vi "UIEH(ver.StateMachine).vi"() -> ()   [LabVIEW 2023]
panel:
  in  "종료":bool
  in  "저장":bool
  in  "분석":bool
  in  "측정":bool
  out "Count":i32
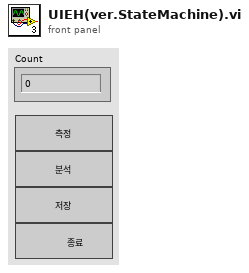
[diagram p1: front panel]
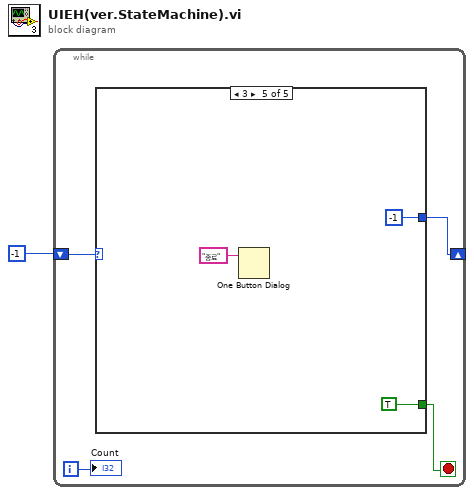
[diagram p0: block diagram]
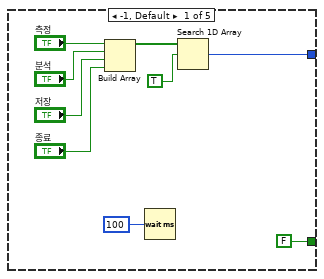
[diagram p2: hidden frame]
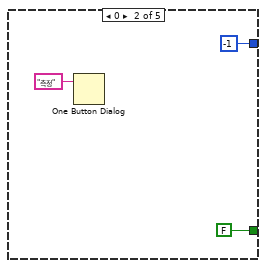
[diagram p3: hidden frame]
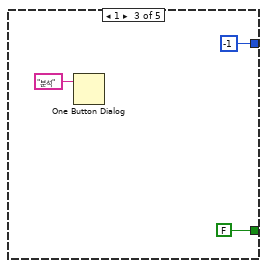
[diagram p4: hidden frame]
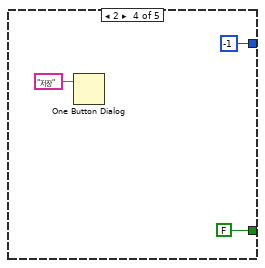
[diagram p5: hidden frame]
diagram:
  n1 = while {
    shift-right: [w2] -> _
    shift-left: -1 -> [w4]
    i -> [w5]
    stop <- w3 stop-if-true
    n2 = case shown="3" w4 {
      tunnel: [FALSE FALSE FALSE FALSE TRUE] -> w3
      tunnel: [w7 -1 ("index of element") -1 ("index of element") -1 ("index of element") -1 ("index of element")] -> w2
      frame -1, Default {
        n3 = Build Array("측정", "분석", "저장", "종료") -> (w8:bool[])
        n4 = Wait (ms)(milliseconds to wait=u32 100) -> ()  [unwired: 1 out]
        n5 = Search 1D Array(1D array=w8, element=TRUE) -> (index of element=w7:i32)  [unwired: 1 in]
      }
      frame 0 {
        n6 = One Button Dialog(message="측정") -> ()  [unwired: 1 in, 1 out]
      }
      frame 1 {
        n7 = One Button Dialog(message="분석") -> ()  [unwired: 1 in, 1 out]
      }
      frame 2 {
        n8 = One Button Dialog(message="저장") -> ()  [unwired: 1 in, 1 out]
      }
      frame 3 {
        n9 = One Button Dialog(message="종료") -> ()  [unwired: 1 in, 1 out]
      }
    }
    "Count" <- w5
  }
